vi "Timer Reset.vi"(9 "Direction":enum8{"either", "false-true", "true-false"}(ring), 10 "Tick Count(Ticks)":u32=40000000, 11 "Start Timer":bool) -> (3 "Timer Running":bool)   [LabVIEW 2017]
doc: "Author: Scott Hannahs <sth@magnet.fsu.edu>\nCopyright 2018 Florida State University, All rights reserved."
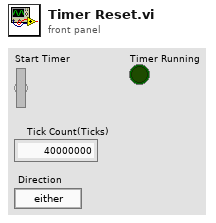
[diagram p1: front panel]
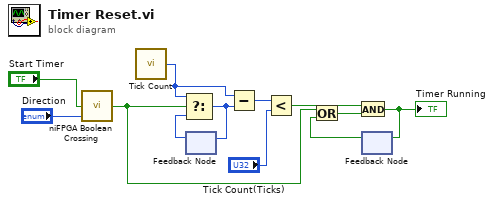
[diagram p0: block diagram]
diagram:
  n1 = call <vilib>:"niFPGA Boolean Crossing.vi"("input"="Start Timer", "direction"="Direction") -> ("crossing"=w1:bool)  [unwired: 7 in]
  n2 = call "Tick Count"() -> ("Tick Count(Ticks)"=w8:u32)
  n3 = feedback #1() -> (w10:u32)  [unwired: 1 in]
  n4 = Select(t=w8, s=w1, f=w10) -> (s? t:f=w9:u32)
  n5 = feedback-in #1(w9) -> ()
  n6 = Subtract(x=w8, y=w9) -> (x-y=w7:u32)
  n7 = Less?(x=w7, y="Tick Count(Ticks)") -> (x < y?=w5:bool)
  n8 = feedback #2() -> (w2:bool)  [unwired: 1 in]
  n9 = Or(x=w1, y=w2) -> (x .or. y?=w3:bool)
  n10 = And(x=w5, y=w3) -> (x .and. y?=w4:bool)
  "Timer Running" <- w4
  n11 = feedback-in #2(w4) -> ()
